vi "Set Heartbeat Producer.vi"(8 "error in":errorcluster, 10 "Heartbeat Production":u32 format="%d ms", 11 "Interactor in":refnum<class "Interactor.lvclass">) -> (0 "error out":errorcluster, 3 "Interactor out":refnum<class "Interactor.lvclass">)   [LabVIEW 2020, in "Interactor.lvlib" / "Interactor.lvclass"]
uses:
  Interactor.lvclass
  Interactor.lvclass/Interactor.ctl
  CANopen Master/CANopen Master.lvclass
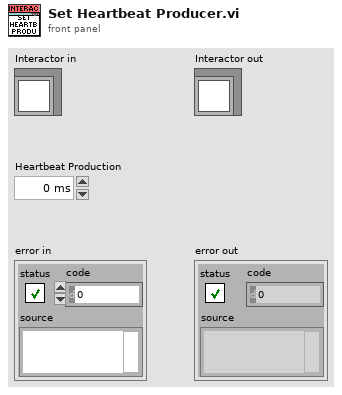
[diagram p1: front panel]
types:
  T1 = cluster{"CAN Task":cluster{"Stop":refnum<user-event>, "Msg Received":refnum<user-event>, "Error":refnum<user-event>}, "NMT":cluster{"Node Discovered":refnum<user-event>}, "Heartbeat Producer":cluster{"Stop":refnum<user-event>, "Error":refnum<user-event>}}
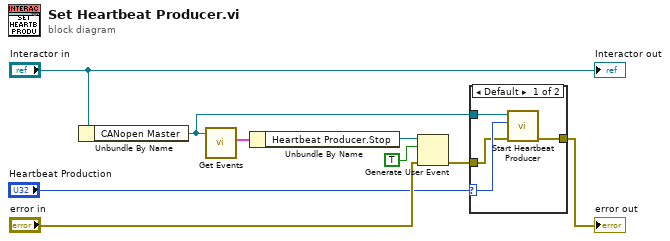
[diagram p0: block diagram]
diagram:
  n1 = Unbundle By Name("Interactor in") -> ("CANopen Master"=w3:refnum<class "CANopen Master.lvclass">)
  n2 = call "Get Events.vi"("CANopen Master in"=w3) -> ("Events"=w7:T1)  [unwired: 9 in, 1 out]
  n3 = Unbundle By Name(w7) -> ("Heartbeat Producer.Stop"=w6:refnum<user-event>)
  n4 = Generate User Event(user event=w6, event data cluster=TRUE ("event data"), error in="error in") -> (error out=w2:errorcluster)  [unwired: 1 in, 1 out]
  n5 = case shown="Default" "Heartbeat Production" {
    selector: "Heartbeat Production" -> [w12 _]
    tunnel: w3 -> [w13 _]
    tunnel: w2 -> [w11 w14]
    tunnel: [w10 w14] -> w1
    frame Default {
      n6 = call "Start Heartbeat Producer.vi"("error in"=w11, "Interval"=w12, "CANopen Master in"=w13) -> ("error out"=w10:errorcluster)  [unwired: 7 in, 1 out]
    }
    frame 0 {
    }
  }
  "error out" <- w1
  "Interactor out" <- "Interactor in"
